vi "Excel File Query.vi"(3 "Filename":string) -> (0 "Excel File?":bool)   [LabVIEW 2013]
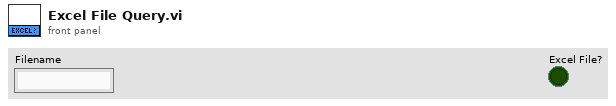
[diagram p1: front panel]
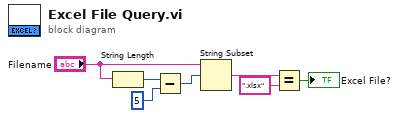
[diagram p0: block diagram]
diagram:
  n1 = String Length(string="Filename") -> (length=w7:i32)
  n2 = Subtract(x=w7, y=5) -> (x-y=w5:i32)
  n3 = String Subset(string="Filename", offset (0)=w5) -> (substring=w3:string)  [unwired: 1 in]
  n4 = Equal?(x=w3, y=".xlsx") -> (x = y?=→"Excel File?":bool)
